vi "CreateTriggerInputNode.vi"(7 "DOM Document":refnum<k20>, 8 "Error In":errorcluster, 11 "Trigger Input Configuration":T1={"Type"=enum."None", "Timeout (ms)"=100, "Delay (ms)"=0, "Digital IO Line (1-14)"=1, "Digital IO Mode"=enum."Falling"}) -> (0 "Error Out":errorcluster, 3 "Trigger Input Node":refnum<k20>)   [LabVIEW 2012]
uses:
  TriggerInputConfiguration.ctl
  TriggerInputType.ctl
  driver/Public/Controls/TriggerMode.ctl
  libs/LV-Utilities/LV-Utilities.lvlib
  driver/Keithley-2602.lvlib
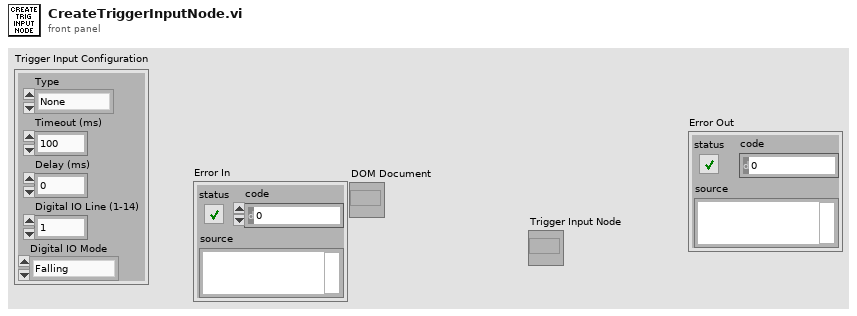
[diagram p1: front panel]
types:
  T1 = typedef "TriggerInputConfiguration.ctl" = cluster{"Type":T2, "Timeout (ms)":u32, "Delay (ms)":u32, "Digital IO Line (1-14)":u8, "Digital IO Mode":T3}
  T2 = typedef "TriggerInputType.ctl" = enum16{"None", "Digital IO", "Bus"}
  T3 = typedef "Keithley-2602.lvlib/TriggerMode.ctl" = enum16{"Falling", "Rising", "Either", "Synchronous"}
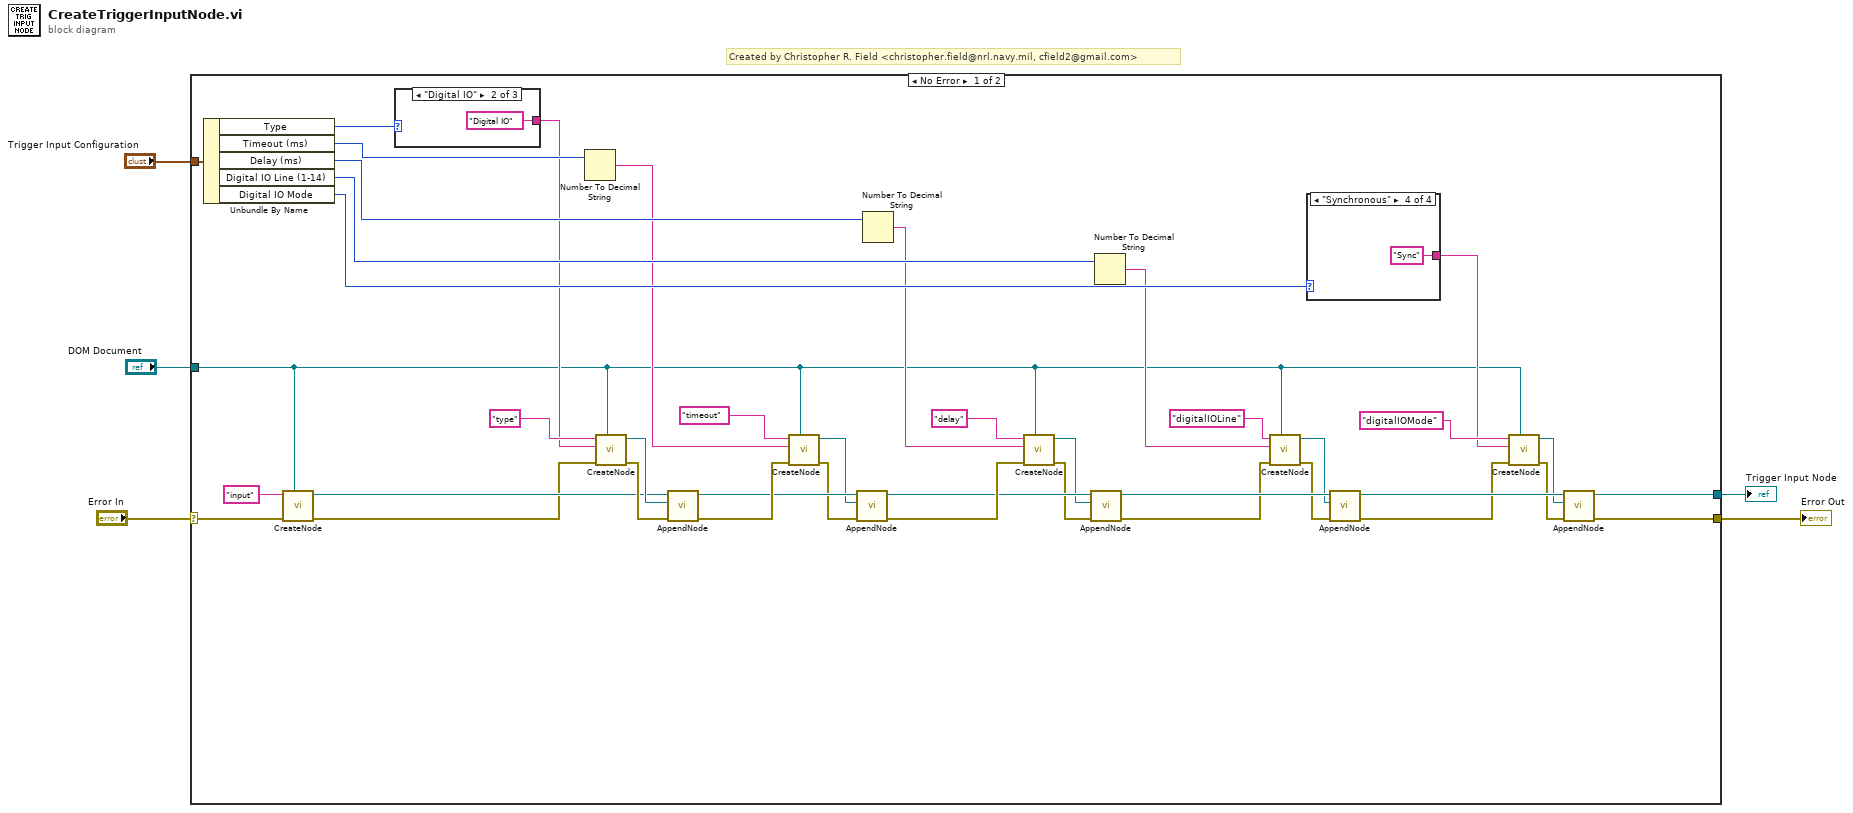
[diagram p0: block diagram]
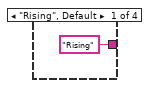
[diagram p2: hidden frame]
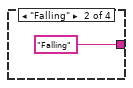
[diagram p3: hidden frame]
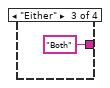
[diagram p4: hidden frame]
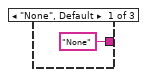
[diagram p5: hidden frame]
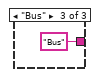
[diagram p6: hidden frame]
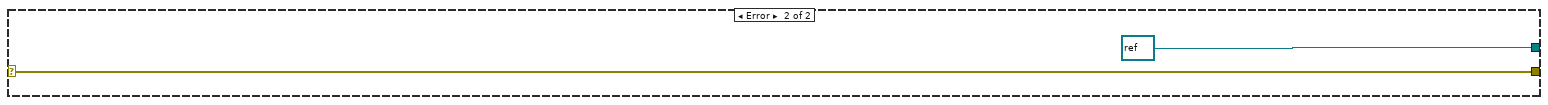
[diagram p7: hidden frame]
diagram:
  # "Created by Christopher R. Field <christopher.field@nrl.navy.mil, cfield2@gmail.com>"
  n1 = case shown="No Error" "Error In" {
    selector: "Error In" -> [w10 w55]
    tunnel: "DOM Document" -> [w8 _]
    tunnel: [w18 refnum<k20> refnum ("Wirings Node 2")] -> w3
    tunnel: [w17 w55] -> w2
    tunnel: "Trigger Input Configuration" -> [w41 _]
    frame No Error {
      n2 = Unbundle By Name(w41) -> ("Type"=w46:T2, "Timeout (ms)"=w42:u32, "Delay (ms)"=w45:u32, "Digital IO Line (1-14)"=w43:u8, "Digital IO Mode"=w44:T3)
      n3 = call "CreateNode.vi"("DOM Document"=w8, "Error In"=w10, "Tag Name"="input") -> ("Error out"=w6:errorcluster, "Node"=w7:refnum<k20>)  [unwired: 7 in]
      n4 = case shown="\"Digital IO\"" w46 {
        tunnel: ["None" "Digital IO" "Bus"] -> w31
        frame "None", Default {
        }
        frame "Digital IO" {
        }
        frame "Bus" {
        }
      }
      n5 = Number To Decimal String(number=w42) -> (decimal integer string=w32:string)  [unwired: 1 in]
      n6 = call "CreateNode.vi"("DOM Document"=w8, "Error In"=w6, "Text"=w31, "Tag Name"="type") -> ("Error out"=w30:errorcluster, "Node"=w29:refnum<k20>)  [unwired: 6 in]
      n7 = call "AppendNode.vi"("Error In"=w30, "Child Node"=w29, "Parent Node In"=w7) -> ("Error Out"=w28:errorcluster, "Parent Node Out"=w27:refnum<k20>)  [unwired: 7 in]
      n8 = call "CreateNode.vi"("DOM Document"=w8, "Error In"=w28, "Text"=w32, "Tag Name"="timeout") -> ("Error out"=w26:errorcluster, "Node"=w25:refnum<k20>)  [unwired: 6 in]
      n9 = call "AppendNode.vi"("Error In"=w26, "Child Node"=w25, "Parent Node In"=w27) -> ("Error Out"=w24:errorcluster, "Parent Node Out"=w23:refnum<k20>)  [unwired: 7 in]
      n10 = Number To Decimal String(number=w45) -> (decimal integer string=w33:string)  [unwired: 1 in]
      n11 = call "CreateNode.vi"("DOM Document"=w8, "Error In"=w24, "Text"=w33, "Tag Name"="delay" ("Text")) -> ("Error out"=w21:errorcluster, "Node"=w22:refnum<k20>)  [unwired: 6 in]
      n12 = call "AppendNode.vi"("Error In"=w21, "Child Node"=w22, "Parent Node In"=w23) -> ("Error Out"=w12:errorcluster, "Parent Node Out"=w20:refnum<k20>)  [unwired: 7 in]
      n13 = Number To Decimal String(number=w43) -> (decimal integer string=w34:string)  [unwired: 1 in]
      n14 = call "CreateNode.vi"("DOM Document"=w8, "Error In"=w12, "Text"=w34, "Tag Name"="digitalIOLine") -> ("Error out"=w13:errorcluster, "Node"=w11:refnum<k20>)  [unwired: 6 in]
      n15 = case shown="\"Synchronous\"" w44 {
        tunnel: ["Rising" "Falling" "Both" "Sync"] -> w35
        frame "Rising", Default {
        }
        frame "Falling" {
        }
        frame "Either" {
        }
        frame "Synchronous" {
        }
      }
      n16 = call "AppendNode.vi"("Error In"=w13, "Child Node"=w11, "Parent Node In"=w20) -> ("Error Out"=w14:errorcluster, "Parent Node Out"=w19:refnum<k20>)  [unwired: 7 in]
      n17 = call "CreateNode.vi"("DOM Document"=w8, "Error In"=w14, "Text"=w35, "Tag Name"="digitalIOMode") -> ("Error out"=w16:errorcluster, "Node"=w15:refnum<k20>)  [unwired: 6 in]
      n18 = call "AppendNode.vi"("Error In"=w16, "Child Node"=w15, "Parent Node In"=w19) -> ("Error Out"=w17:errorcluster, "Parent Node Out"=w18:refnum<k20>)  [unwired: 7 in]
    }
    frame Error {
    }
  }
  "Trigger Input Node" <- w3
  "Error Out" <- w2
